vi "case_structure.vi"() -> ()   [LabVIEW 2015]
panel:
  in  "stop":bool
  in  "Ring":u16(ring) items=["ADD", "SUB", "MUL", "DIV"]
  in  "Int Choice":i32
  in  "String choice":string
  out "RESULT":dbl
  in  "OP2":dbl
  in  "OP1":dbl
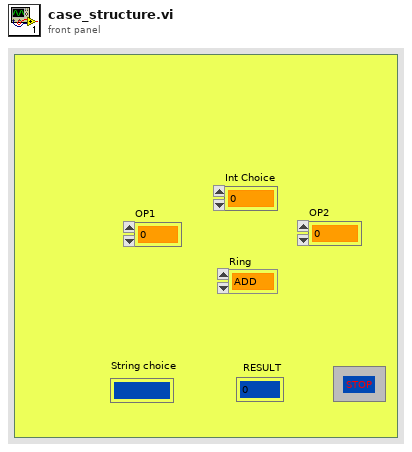
[diagram p1: front panel]
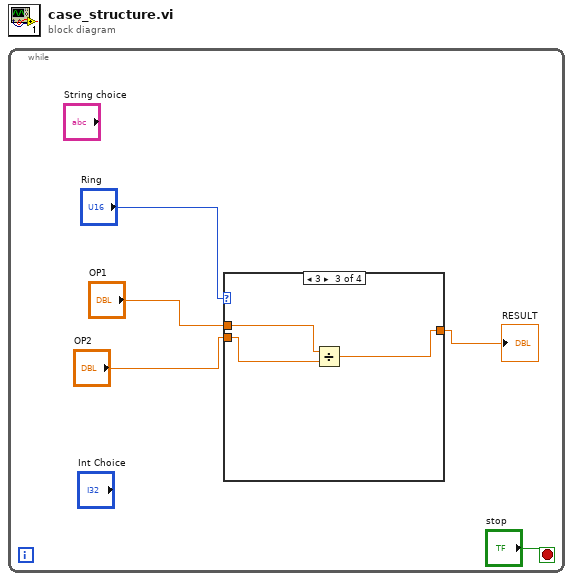
[diagram p0: block diagram]
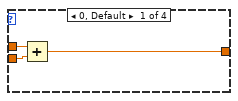
[diagram p2: hidden frame]
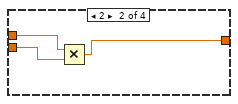
[diagram p3: hidden frame]
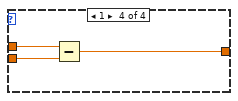
[diagram p4: hidden frame]
diagram:
  n1 = while {
    stop <- "stop" stop-if-true
    n2 = case shown="3" "Ring" {
      tunnel: "OP1" -> [w8 w11 w14 w17]
      tunnel: "OP2" -> [w7 w10 w13 w16]
      tunnel: [w6 w9 w12 w15] -> w3
      frame 0, Default {
        n3 = Add(x=w8, y=w7) -> (x+y=w6:dbl)
      }
      frame 2 {
        n4 = Multiply(x=w11, y=w10) -> (x*y=w9:dbl)
      }
      frame 3 {
        n5 = Divide(x=w14, y=w13) -> (x/y=w12:dbl)
      }
      frame 1 {
        n6 = Subtract(x=w17, y=w16) -> (x-y=w15:dbl)
      }
    }
    "RESULT" <- w3
  }
